vi "GrowArray.vi"(9 "grow":i32, 10 "index":i32, 11 "PipeData in":refnum<class "StreamData.lvclass">) -> (3 "PipeData out":refnum<class "StreamData.lvclass">)   [LabVIEW 2017, in "Stream-t'WPI_EncoderType.ctl'.lvlib" / "StreamData.lvclass"]
uses:
  <extravilib>/ChannelInstances/Stream-t'WPI_EncoderType.ctl'/StreamData.lvclass
  <extravilib>/ChannelInstances/Stream-t'WPI_EncoderType.ctl'/StreamData.lvclass/StreamData.ctl
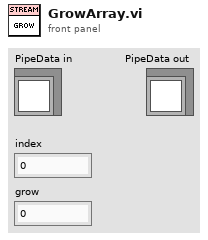
[diagram p1: front panel]
types:
  T1 = typedef "WPI_EncoderType.ctl" = enum16{"1x", "2x", "4x"}
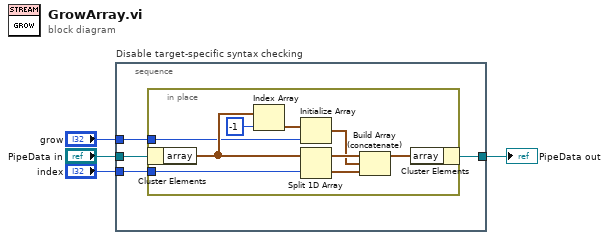
[diagram p0: block diagram]
diagram:
  n1 = stacked-sequence "Disable target-specific syntax checking" {
    tunnel: [w8] -> w4
    tunnel: "PipeData in" -> [w7]
    tunnel: "index" -> [w6]
    tunnel: "grow" -> [w5]
    frame #0 {
      n2 = in-place {
        in-place-border: w6 -> [w16]
        in-place-border: w5 -> [w14]
        n3 = in-place-cluster #1(w7) -> ("array"=w17:cluster{"element":T1}[])
        n4 = Index Array(array=w17, index=-1) -> (element=w10:cluster{"element":T1})
        n5 = Initialize Array(w10, w14) -> (w9:cluster{"element":T1}[])
        n6 = Split 1D Array(array=w17, index=w16) -> (first subarray=w13:cluster{"element":T1}[], second subarray=w12:cluster{"element":T1}[])
        n7 = Build Array (concatenate)(w13, w9, w12) -> (w15:cluster{"element":T1}[])
        n8 = in-place-cluster #1("array"=w15) -> (w8:refnum<class "StreamData.lvclass">)
      }
    }
  }
  "PipeData out" <- w4
